vi "CloseFAGraph.vi"(8 "error in (no error)":errorcluster caption="entrée d'erreur (pas d'erreur)", 9 "UpdtGphConf":bool, 10 "GraphIndexArr":i32[](array[numeric]), 11 "Interface en entrée":refnum<class "Interface.lvclass"> caption="DNL_LabVIEW Object in") -> (0 "error out":errorcluster caption="sortie d'erreur", 3 "Interface en sortie":refnum<class "Interface.lvclass"> caption="DNL_LabVIEW Object out")   [LabVIEW 2012, in "Interface.lvclass"]
uses:
  Interface.lvclass
  Interface.lvclass/Interface.ctl
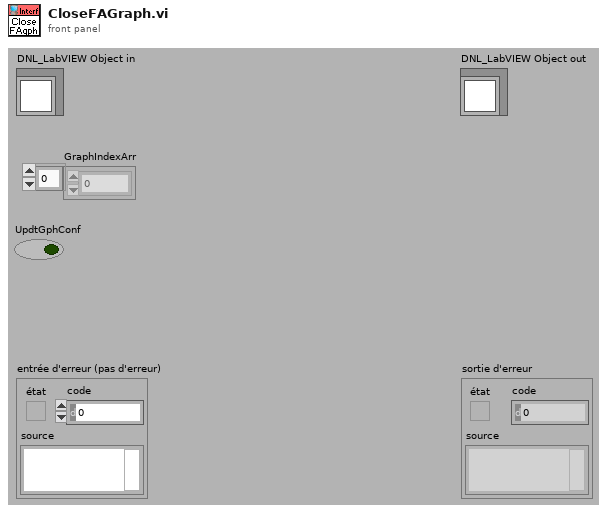
[diagram p1: front panel]
types:
  T1 = typedef "Interface.lvclass/CurveSetup.ctl" = cluster{"CurveName":string, "YParam":string, "XParam":string, "ZParam ":string, "GroupName":string, "LinWdth":u8, "PntCol":u32, "LinCol":u32, "LablFor":u8, "XScale":u32, "YScale":u32, "Interpol":u8, "DisplayName":string, "FillType":i16, "LineStyle":u8, "PntStyle":u8, "BarTyp":u8, "GraphIndex":i32, "Visible":bool, "XScaleName":string, "YScaleName":string, "XYGraph_Ref":refnum<vi>, "Data Only":bool, "DataQ Ref":refnum<queue>, "XParQ Ref":refnum<queue>, "XParamInd":i32, "ScanInd":i32}
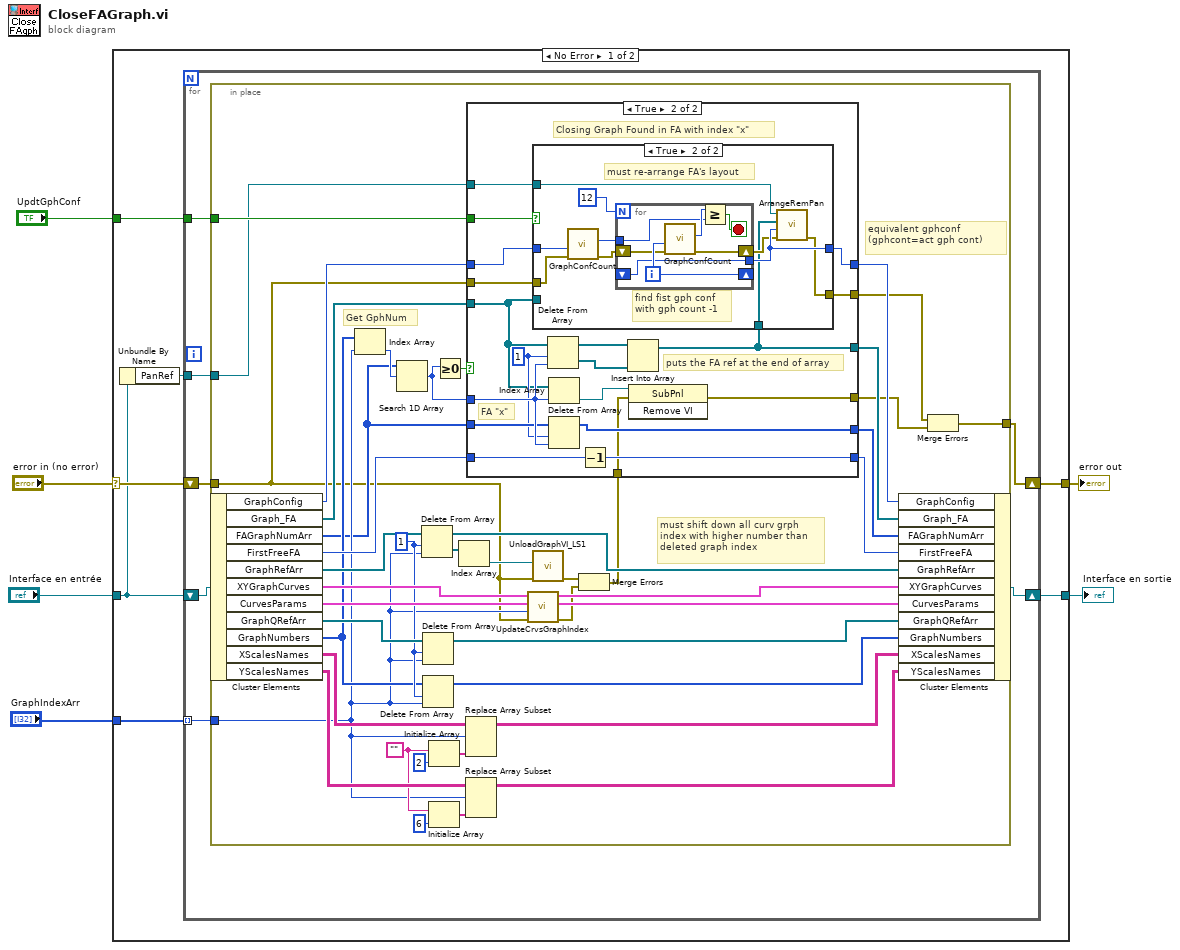
[diagram p0: block diagram]
diagram:
  n1 = case shown="No Error" "error in (no error)" {
    selector: "error in (no error)" -> [w12 w108]
    tunnel: [w10 w108] -> w5
    tunnel: [w11 w107] -> w3
    tunnel: "Interface en entrée" -> [w8 w107]
    tunnel: "GraphIndexArr" -> [w13 _]
    tunnel: "UpdtGphConf" -> [w9 _]
    frame No Error {
      n2 = Unbundle By Name(w8) -> ("PanRef"=w7:refnum<vi>)
      n3 = for {
        tunnel: w13 -> [w20] mode=indexing
        shift-right: [w17] -> w10
        shift-left: w12 -> [w18]
        shift-right: [w16] -> w11
        shift-left: w8 -> [w19]
        tunnel: w9 -> [w15]
        tunnel: w7 -> [w14]
        n4 = in-place {
          in-place-border: w20 -> [w29]
          in-place-border: w18 -> [w26]
          in-place-border: [w23] -> w17
          in-place-border: w15 -> [w35]
          in-place-border: w14 -> [w22]
          w51 = ""
          w34 = 1 ("longueur")
          # "Get GphNum"
          # "equivalent gphconf\n(gphcont=act gph cont)"
          # "must shift down all curv grph\nindex with higher number than\ndeleted graph index"
          n5 = in-place-cluster #1(w19) -> ("GraphConfig"=w44:i32, "Graph_FA"=w49:refnum<vi>[], "FAGraphNumArr"=w28:i32[], "FirstFreeFA"=w47:u8, "GraphRefArr"=w63:refnum<vi>[], "XYGraphCurves"=w40:cluster{"Tableau":i32[]}[], "CurvesParams"=w38:T1[], "GraphQRefArr"=w42:refnum<queue>[], "GraphNumbers"=w31:i32[], "XScalesNames"=w59:string[][], "YScalesNames"=w54:string[][])
          n6 = Index Array(array=w31, index=w29) -> (element=w30:i32)
          n7 = Search 1D Array(1D array=w28, element=w30) -> (index of element=w32:i32)  [unwired: 1 in]
          n8 = Delete From Array(array=w63, length=w34, index=w29) -> (deleted portion=w61:refnum<vi>[], array with subset deleted=w62:refnum<vi>[])
          n9 = Delete From Array(array=w42, length=w34, index=w29) -> (array with subset deleted=w41:refnum<queue>[])  [unwired: 1 out]
          n10 = Delete From Array(array=w31, length=w34, index=w29) -> (array with subset deleted=w33:i32[])  [unwired: 1 out]
          n11 = Initialize Array(w51, 2 ("taille de la dimension")) -> (w57:string[])
          n12 = Initialize Array(w51, 6 ("taille de la dimension")) -> (w56:string[])
          n13 = Greater Or Equal To 0?(x=w32) -> (x >= 0?=w50:bool)
          n14 = Index Array(array=w61) -> (element=w60:refnum<vi>)  [unwired: 1 in]
          n15 = Replace Array Subset(array=w59, new element=w57, index (row)=w29) -> (w52:string[][])  [unwired: 1 in]
          n16 = Replace Array Subset(array=w54, new element=w56, index (row)=w29) -> (w53:string[][])  [unwired: 1 in]
          n17 = call "UpdateCrvsGraphIndex.vi"("error in (no error)"=w26, "DelGraphIndex"=w29, "CurvesParams"=w38, "XYGraphCurves"=w40) -> ("error out"=w36:errorcluster, "CurvesParams Out"=w37:T1[], "XYGraphCrvsOut"=w39:cluster{"Tableau":i32[]}[])  [unwired: 5 in]
          n18 = call "UnloadGraphVI_LS1.vi"("ErrorIn(No Error)"=w26, "GraphRef"=w60) -> ("sortie d'erreur"=w48:errorcluster)  [unwired: 9 in]
          n19 = Merge Errors(w48, w36) -> (w21:errorcluster)
          n20 = case shown="True" w50 {
            tunnel: w32 -> [_ w78]
            tunnel: w49 -> [w67 w74]
            tunnel: w47 -> [w68 w86]
            tunnel: [w68 w85] -> w46
            tunnel: [w64 w84] -> w24
            tunnel: [w67 w69] -> w45
            tunnel: w44 -> [w66 w80]
            tunnel: [w66 w81] -> w43
            tunnel: w35 -> [_ w79]
            tunnel: w28 -> [w65 w77]
            tunnel: [w65 w75] -> w27
            tunnel: w26 -> [w64 w71]
            tunnel: [w64 w73] -> w25
            tunnel: w22 -> [_ w72]
            tunnel: w21 -> [_ w70]
            frame False {
              # "closing free floating graph"
            }
            frame True {
              w76 = 1 ("longueur")
              # "puts the FA ref at the end of array"
              # "FA \"x\""
              # "Closing Graph Found in FA with index \"x\""
              n21 = Delete From Array(array=w74, length=w76, index=w78) -> (deleted portion=w82:refnum<vi>[], array with subset deleted=w83:refnum<vi>[])
              n22 = Index Array(array=w74, index=w78) -> (element=w87:refnum<vi>)
              n23 = Delete From Array(array=w77, length=w76, index=w78) -> (array with subset deleted=w75:i32[])  [unwired: 1 out]
              n24 = Decrement(x=w86) -> (x-1=w85:u8)
              n25 = Insert Into Array(array=w83, new element=w82) -> (w69:refnum<vi>[])  [unwired: 1 in]
              n26 = case shown="True" w79 {
                tunnel: w80 -> [w89 w99]
                tunnel: [w89 w94] -> w81
                tunnel: w74 -> [_ _]
                tunnel: w71 -> [w88 w95]
                tunnel: [w88 w92] -> w73
                tunnel: w72 -> [_ w91]
                tunnel: w69 -> [_ w90]
                frame False {
                }
                frame True {
                  # "must re-arrange FA's layout"
                  # "find fist gph conf\nwith gph count -1"
                  n27 = call "GraphConfCount.vi"("error in (no error)"=w95, "Configuration"=w99) -> ("error out"=w97:errorcluster, "GraphCount"=w98:i32)  [unwired: 8 in]
                  n28 = for {
                    N: 12 -> [_]
                    tunnel: w98 -> [w100]
                    shift-right: [w106] -> _
                    shift-left: _ -> [w105]
                    tunnel: [w105] -> w94
                    shift-right: [w102] -> w93
                    shift-left: w97 -> [w104]
                    i -> [w106]
                    stop <- w103 stop-if-true
                    n29 = call "GraphConfCount.vi"("error in (no error)"=w104, "Configuration"=w106) -> ("error out"=w102:errorcluster, "GraphCount"=w101:i32)  [unwired: 8 in]
                    n30 = Greater Or Equal?(x=w101, y=w100) -> (x >= y?=w103:bool)
                  }
                  n31 = call "ArrangeRemPan.vi"("error in (no error)"=w93, "Configuration"=w94, "FARefArr"=w90, "PanRef"=w91) -> ("error out"=w92:errorcluster)  [unwired: 5 in, 2 out]
                }
              }
              n32 = invoke class="SubPnl" method="Remove VI"(reference=w87, error in=w70) -> (error out=w84:errorcluster)  [unwired: 1 in, 2 out]
            }
          }
          n33 = in-place-cluster #1("GraphConfig"=w43, "Graph_FA"=w45, "FAGraphNumArr"=w27, "FirstFreeFA"=w46, "GraphRefArr"=w62, "XYGraphCurves"=w39, "CurvesParams"=w37, "GraphQRefArr"=w41, "GraphNumbers"=w33, "XScalesNames"=w52, "YScalesNames"=w53) -> (w16:refnum<class "Interface.lvclass">)
          n34 = Merge Errors(w25, w24) -> (w23:errorcluster)
        }
      }
    }
    frame Error {
    }
  }
  "error out" <- w5
  "Interface en sortie" <- w3
